vi "Module Identities.vi"(8 "error in (no error)":errorcluster, 11 "GUI Manager Module in":refnum<class "GUI Manager Module.lvclass">) -> (0 "error out":errorcluster, 2 "Identities":refnum<class "Identity.lvclass">[](array[class]), 3 "GUI Manager Module out":refnum<class "GUI Manager Module.lvclass">)   [LabVIEW 2020, in "VolatusGUI.lvlib" / "GUI Manager Module.lvclass"]
uses:
  GUI Manager Module.lvclass
  Volatus/Identity/Identity.lvclass
  GUI Manager Module.lvclass/GUI Manager Module.ctl
  GUI Manager Identity/GUI Manager Identity.lvclass
  GUI Identity/GUI Identity.lvclass
  C:/dev/lv20CE/relink/lv-volatus/VolatusGUI/GUI Manager Identity/GUI Manager Identity.lvclass
  C:/dev/lv20CE/relink/lv-volatus/Volatus/Identity/Identity.lvclass
  C:/dev/lv20CE/relink/lv-volatus/VolatusGUI/GUI Identity/GUI Identity.lvclass
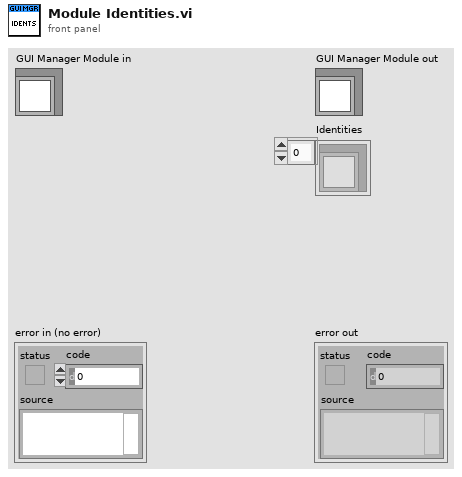
[diagram p1: front panel]
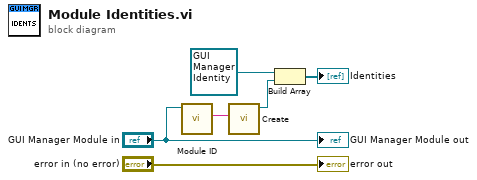
[diagram p0: block diagram]
diagram:
  n1 = call-dynamic "Module ID.vi"("GUI Manager Module in"="GUI Manager Module in") -> ("Module ID"=w4:string)  [unwired: 10 in]
  n2 = call "Create.vi"("Module ID"=w4) -> ("GUI Identity out"=w3:refnum<class "GUI Identity.lvclass">)  [unwired: 10 in]
  n3 = Build Array(refnum<class "GUI Manager Identity.lvclass"> refnum ("VolatusGUI:GUI Manager Identity.lvclass"), w3) -> (→"Identities":refnum<class "Identity.lvclass">[])
  "error out" <- "error in (no error)"
  "GUI Manager Module out" <- "GUI Manager Module in"
